vi "axex_save_file_office16.vi"(7 "force operation (ignore error in) (True)":bool=TRUE, 8 "error in":errorcluster, 9 "file overwrite prompt (True)":bool=TRUE, 10 "file path (no path)":path, 11 "AX Excel instance in":T1) -> (0 "error out":errorcluster, 3 "AX Excel instance out":T1)   [LabVIEW 2020, in "AX Excel.lvlib"]
doc: "Note: Office 2016 version - disabled SaveAs() method, excel file must be opened, not created!\n\nCall this to save unsaved changes in given file.\nIf current workbook is new workbook (not loaded from file) the file path must be entered.\nIf you want to change the save path from implicit (the path from which it was opened), you can enter new path."
uses:
  AX Excel.lvlib
  axex_instance.ctl
  <vilib>/Utility/error.llb/Error Cluster From Error Code.vi
  <vilib>/ErrorRing/Error Ring.xnode
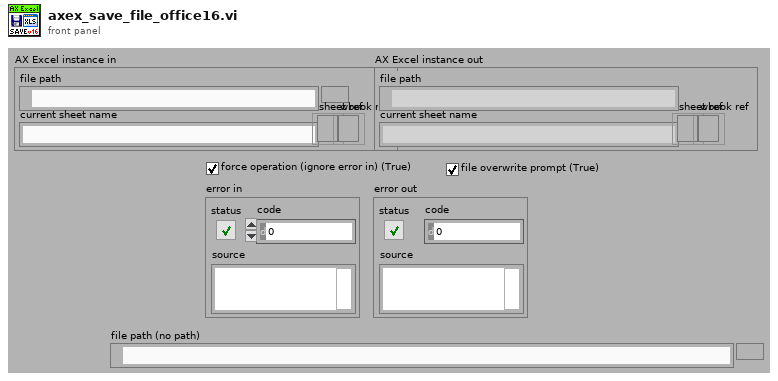
[diagram p1: front panel]
types:
  T1 = typedef "AX Excel.lvlib/axex_instance.ctl" = cluster{"file path":path, "current sheet name":string, "sheet ref":refnum<k7>, "wbook ref":refnum<k7>}
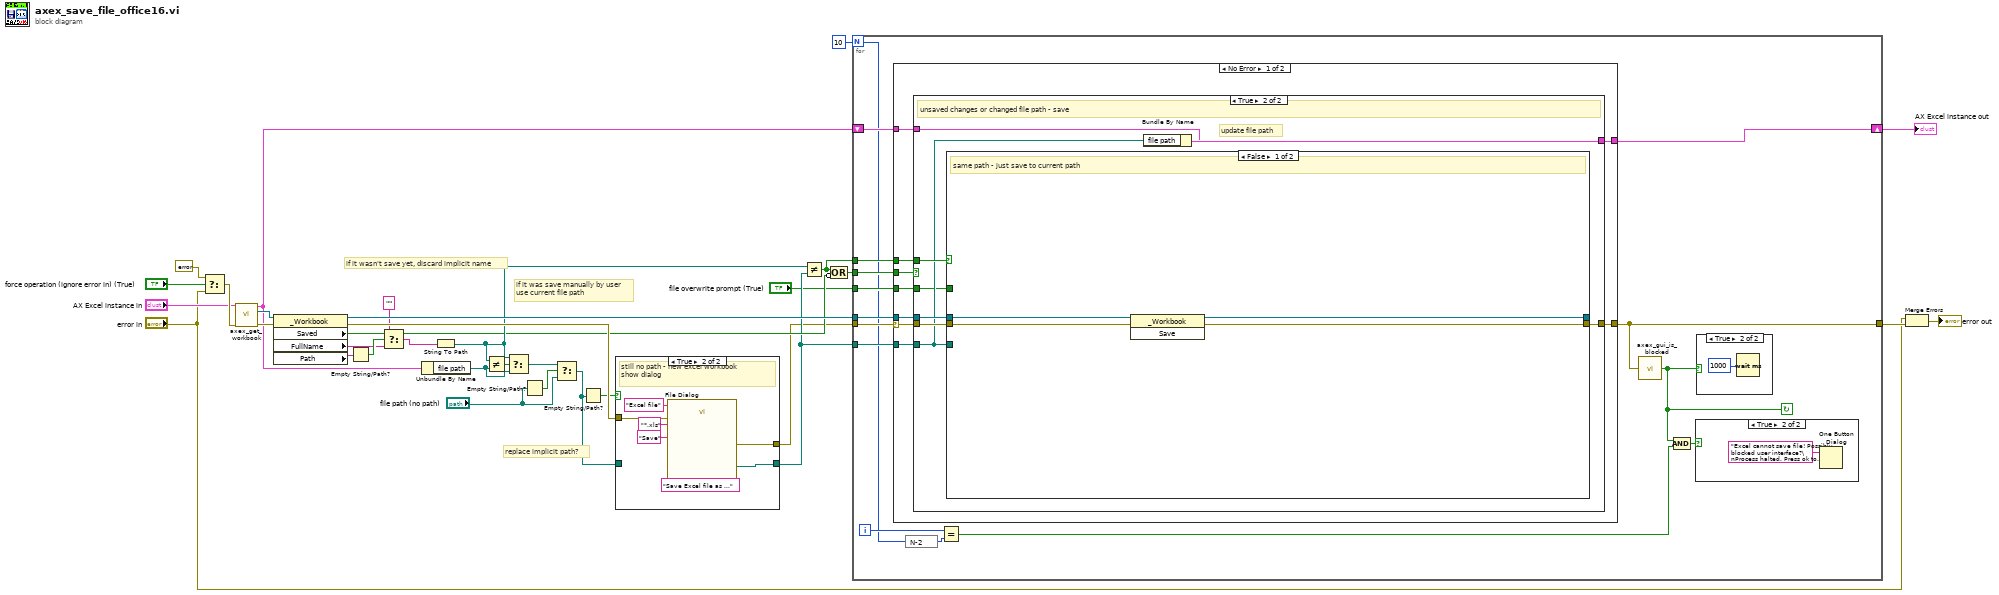
[diagram p0: block diagram]
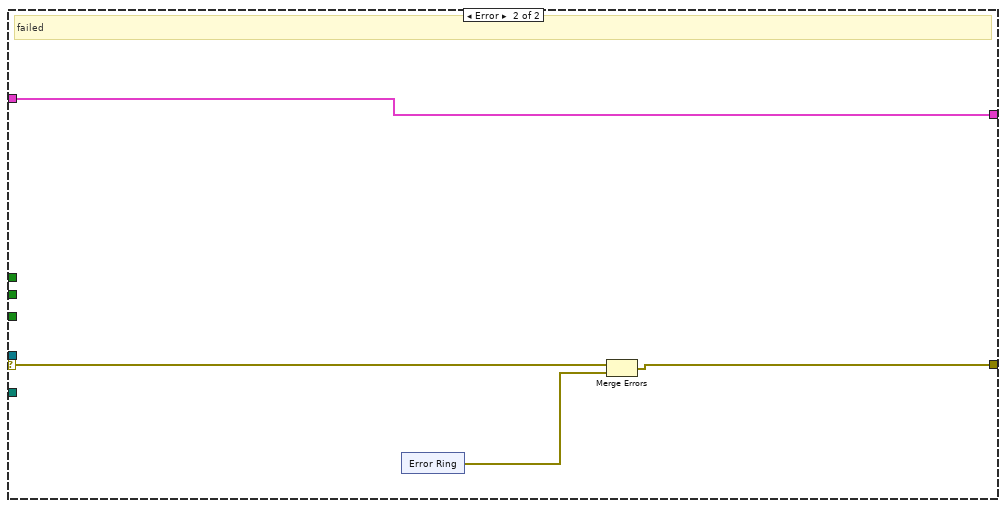
[diagram p6: hidden frame]
diagram:
  # "if it was save manually by user\nuse current file path"
  # "if it wasn't save yet, discard implicit name"
  # "replace implicit path?"
  n1 = Select(t=errorcluster {"status"=FALSE, "code"=0, "source"=""}, s="force operation (ignore error in) (True)", f="error in") -> (s? t:f=w31:errorcluster)
  n2 = call "axex_get_workbook.vi"("error in"=w31, "AX Excel instance in"="AX Excel instance in") -> ("error out"=w33:errorcluster, "excel workbook"=w26:refnum<k7>, "AX Excel instance out"=w9:T1)  [unwired: 7 in]
  n3 = property class="_Workbook"(reference=w26, error in=w33) -> (reference out=w32:refnum<k7>, error out=w20:errorcluster, "Saved"=w15:bool, "FullName"=w5:string, "Path"=w7:string)
  n4 = Empty String/Path?(string/path=w7) -> (empty?=w6:bool)
  n5 = Select(t="", s=w6, f=w5) -> (s? t:f=w3:string)
  n6 = Unbundle By Name(w9) -> ("file path"=w22:path)
  n7 = String To Path(string=w3) -> (path=w16:path)
  n8 = Not Equal?(x=w16, y=w22) -> (x != y?=w23:bool)
  n9 = Select(t=w16, s=w23, f=w22) -> (s? t:f=w21:path)
  n10 = Empty String/Path?(string/path="file path (no path)") -> (empty?=w25:bool)
  n11 = Select(t=w21, s=w25, f="file path (no path)") -> (s? t:f=w18:path)
  n12 = Empty String/Path?(string/path=w18) -> (empty?=w19:bool)
  n13 = case shown="True" w19 {
    tunnel: w20 -> [w35 w41]
    tunnel: [w35 w40] -> w12
    tunnel: [w34 w39] -> w13
    tunnel: w18 -> [w34 _]
    frame False {
      # "we have path - do nothing"
    }
    frame True {
      # "still no path - new excel workbook\nshow dialog"
      n14 = call "File Dialog"("prompt"="Save Excel file as ...", "button label"="Save", "error in"=w41, "pattern (all files)"="*.xls", "pattern label"="Excel file") -> ("selected path"=w39:path, "error out"=w40:errorcluster)  [unwired: 7 in, 2 out]
    }
  }
  n15 = Not Equal?(x=w16, y=w13) -> (x != y?=w14:bool)
  n16 = Compound Arithmetic op=OR(w14, invert w15) -> (w17:bool)
  n17 = for {
    N: 10 -> [w46]
    tunnel: w32 -> [w57]
    tunnel: w17 -> [w56]
    tunnel: w14 -> [w55]
    tunnel: w13 -> [w54]
    tunnel: w12 -> [w53]
    tunnel: [w48] -> w11
    tunnel: "file overwrite prompt (True)" -> [w50]
    shift-right: [w52] -> w10
    shift-left: w9 -> [w51]
    i -> [w47]
    stop <- w43 continue-if-true
    n18 = case shown="No Error" w53 {
      selector: w53 -> [w64 w88]
      tunnel: w57 -> [w68 _]
      tunnel: w56 -> [w67 _]
      tunnel: w55 -> [w66 _]
      tunnel: w54 -> [w65 _]
      tunnel: [w63 w86] -> w48
      tunnel: [w62 w85] -> w52
      tunnel: w51 -> [w61 w85]
      tunnel: w50 -> [w60 _]
      frame No Error {
        n19 = case shown="True" w67 {
          tunnel: w68 -> [_ w78]
          tunnel: w64 -> [w70 w77]
          tunnel: w66 -> [_ w76]
          tunnel: w65 -> [_ w74]
          tunnel: [w70 w72] -> w63
          tunnel: [w69 w75] -> w62
          tunnel: w61 -> [w69 w73]
          tunnel: w60 -> [_ w71]
          frame False {
            # "no changes - no save"
          }
          frame True {
            # "update file path"
            # "unsaved changes or changed file path - save"
            n20 = case shown="False" w76 {
              tunnel: w77 -> [w82 w84]
              tunnel: w78 -> [w81 w83]
              tunnel: [w80 w84] -> w72
              tunnel: [w79 w83] -> _
              tunnel: w74 -> [_ _]
              tunnel: w71 -> [_ _]
              frame False {
                # "same path - just save to current path"
                n21 = invoke class="_Workbook" method="Save"(reference=w81, error in=w82) -> (reference out=w79:refnum<k7>, error out=w80:errorcluster)  [unwired: 1 in, 1 out]
              }
              frame True {
                # "removed because of Office 2016 fucked up SaveAs method"
                # "different path - save as"
              }
            }
            n22 = Bundle By Name(cluster=w73, "file path"=w74) -> (w75:T1)
          }
        }
      }
      frame Error {
        # "failed"
        n23 = xnode "Error Ring"() -> ("error out"=w87:errorcluster)
        n24 = Merge Errors(w88, w87) -> (w86:errorcluster)
      }
    }
    n25 = expression code="N-2"(w46) -> (w45:i32)
    n26 = Equal?(x=w47, y=w45) -> (x = y?=w44:bool)
    n27 = call "axex_gui_is_blocked.vi"("error in"=w48) -> ("gui blocked?"=w43:bool)
    n28 = Compound Arithmetic op=AND(w43, w44) -> (w49:bool)
    n29 = case shown="True" w49 {
      frame False {
      }
      frame True {
        n30 = One Button Dialog(message="Excel cannot save file! Possibly blocked user interface?\nProcess halted. Press ok to retry.") -> ()  [unwired: 1 in, 1 out]
      }
    }
    n31 = case shown="True" w43 {
      frame False {
      }
      frame True {
        n32 = Wait (ms)(milliseconds to wait=u32 1000) -> ()  [unwired: 1 out]
      }
    }
  }
  "AX Excel instance out" <- w10
  n33 = Merge Errors("error in", w11) -> (→"error out":errorcluster)
